vi "Test Next Shows Next Test to Run in Flat Test Suite.vi"(8 "error in (no error)":errorcluster, 11 "Test Case In":refnum<class "Test Suite Enumeration Test.lvclass">) -> (0 "error out":errorcluster, 3 "Test Case Out":refnum<class "Test Suite Enumeration Test.lvclass">)   [LabVIEW 2020, in "Test Suite Enumeration Test.lvclass"]
uses:
  Test Suite Enumeration Test.lvclass
  Test Suite Enumeration Test.lvclass/Test Suite Enumeration Test.ctl
  Test Doubles/Test Case Test Double Child/Light Test Case Double.lvclass
  6b7f3171-a55a-44cc-8f9a-4994299db920.vi
  source/LUnit Test Suite.lvclass
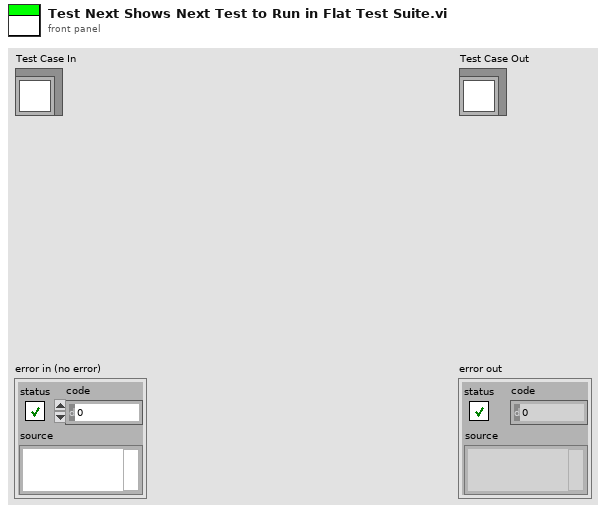
[diagram p1: front panel]
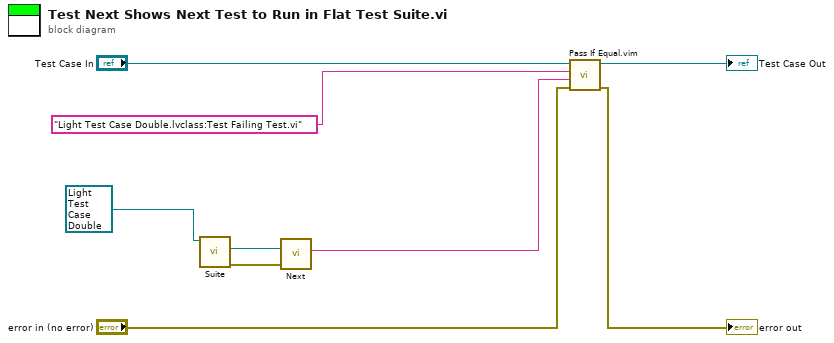
[diagram p0: block diagram]
diagram:
  n1 = call-dynamic "Suite.vi"("LUnit Test Case In"=refnum<class "Light Test Case Double.lvclass"> refnum ("Light Test Case Double.lvclass")) -> ("error out"=w3:errorcluster, "LUnit Test Suite Out"=w5:refnum<class "LUnit Test Suite.lvclass">)  [unwired: 8 in, 1 out]
  n2 = call "Next.vi"("error in (no error)"=w3, "LUnit Test Suite In"=w5) -> ("Next Runnable"=w2:string)  [unwired: 7 in, 2 out]
  n3 = call "Pass If Equal.vim"("error in (no error)"="error in (no error)", "Actual"=w2, "Expected"="Light Test Case Double.lvclass:Test Failing Test.vi" ("Name"), "LUnit Test Case In"="Test Case In") -> ("error out"=→"error out":errorcluster, "LUnit Test Case Out"=→"Test Case Out":refnum<class "Test Suite Enumeration Test.lvclass">)  [unwired: 6 in]
